vi "ADCP_read_parameter_from_serial_port_Test.vi"() -> ()   [LabVIEW 2017]
uses:
  Classes/ADCP.lvclass
panel:
  in  "Stop Application":bool
  out "Parameter Value":string
  in  "Parameter to monitor":string(combo)
  in  "Symbol File Path":path
  in  "ADCP Session Parameters":T1
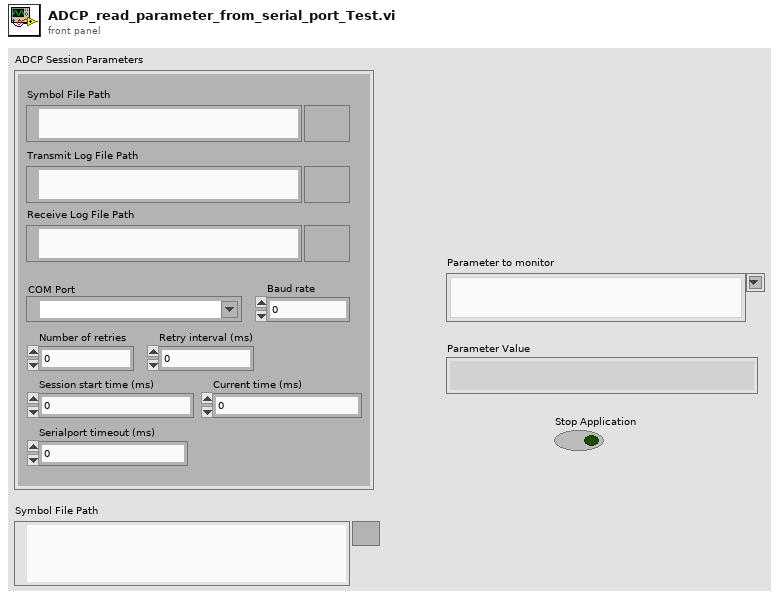
[diagram p1: front panel]
types:
  T1 = cluster{"Symbol File Path":path, "Transmit Log File Path":path, "Receive Log File Path":path, "COM Port":refnum<visa-resource-name>, "Baud rate":u32, "Number of retries":u16, "Retry interval (ms)":u16, "Session start time (ms)":u32, "Current time (ms)":u32, "Serialport timeout (ms)":u32}
  T2 = typedef "ADCP.lvclass/ADCP_Packet_Info.ctl" = cluster{"Priority":enum16{"LOW", "HIGH"}, "Type":enum16{"Data", "Connection Management", "Remote Request", "Error and status", "INVALID"}, "Node ID":i32, "Frame ID":i32, "Checksum valid ?":bool, "Current time (ms)":u32}
  T3 = enum16{"Data", "Connection Management", "Remote Request", "Error and status", "INVALID"}
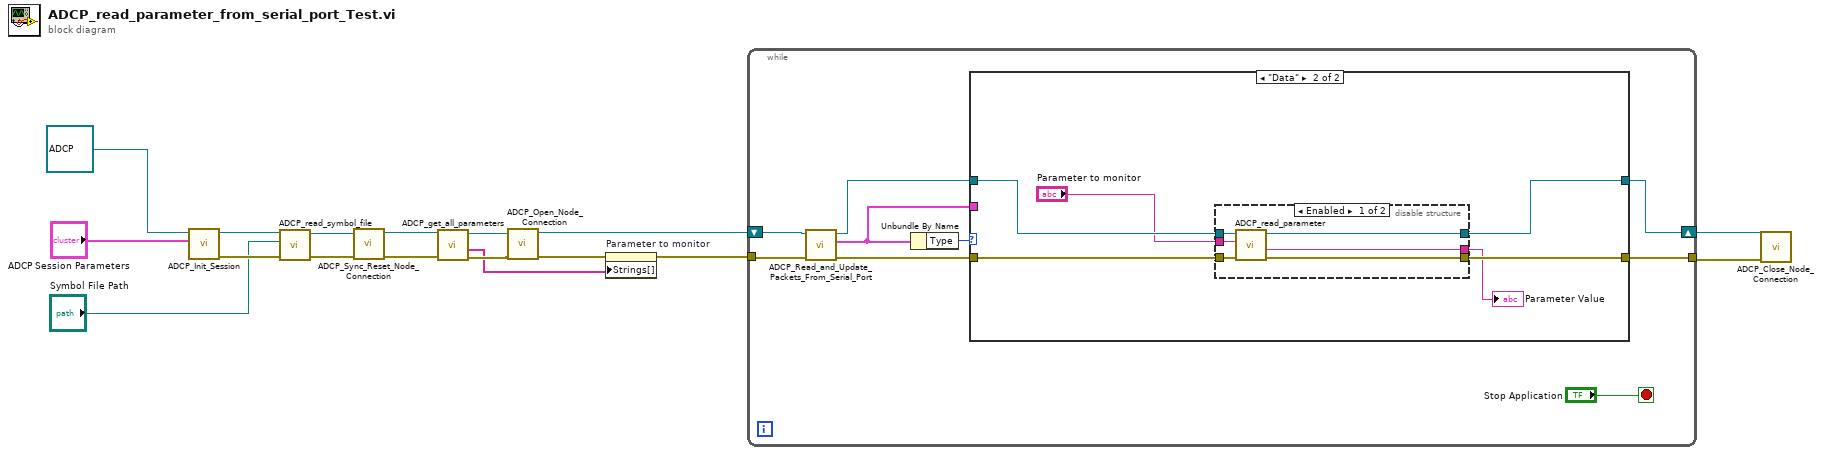
[diagram p0: block diagram]
diagram:
  n1 = call "ADCP_Init_Session.vi"("ADCP Session Parameters"="ADCP Session Parameters", "ADCP in"=refnum<class "ADCP.lvclass"> refnum) -> ("error out"=w15:errorcluster, "ADCP out"=w16:refnum<class "ADCP.lvclass">)  [unwired: 8 in]
  n2 = call "ADCP_read_symbol_file.vi"("error in (no error)"=w15, "Symbol File Path"="Symbol File Path", "ADCP in"=w16) -> ("error out"=w2:errorcluster, "ADCP out"=w4:refnum<class "ADCP.lvclass">)  [unwired: 5 in, 2 out]
  n3 = call "ADCP_Sync_Reset_Node_Connection.vi"("error in (no error)"=w2, "ADCP In"=w4) -> ("error out"=w1:errorcluster, "ADCP Out"=w3:refnum<class "ADCP.lvclass">)  [unwired: 8 in]
  n4 = call "ADCP_get_all_parameters.vi"("error in (no error)"=w1, "ADCP In"=w3) -> ("error out"=w12:errorcluster, "Parameter names"=w9:string[], "ADCP Out"=w13:refnum<class "ADCP.lvclass">)  [unwired: 6 in, 1 out]
  n5 = call "ADCP_Open_Node_Connection.vi"("error in (no error)"=w12, "ADCP In"=w13) -> ("error out"=w10:errorcluster, "ADCP Out"=w11:refnum<class "ADCP.lvclass">)  [unwired: 8 in]
  n6 = property on="Parameter to monitor" class="CmbBox"(error in=w10, "Strings[]"=w9) -> (error out=w8:errorcluster)  [unwired: 1 in, 1 out]
  n7 = while {
    tunnel: w8 -> [w25]
    shift-right: [w20] -> w7
    shift-left: w11 -> [w26]
    tunnel: [w19] -> w6
    stop <- "Stop Application" stop-if-true
    n8 = call "ADCP_Read_and_Update_Packets_From_Serial_Port.vi"("error in (no error)"=w25, "ADCP In"=w26) -> ("error out"=w22:errorcluster, "Packet Info"=w21:T2, "ADCP out"=w23:refnum<class "ADCP.lvclass">)  [unwired: 6 in, 1 out]
    n9 = Unbundle By Name(w21) -> ("Type"=w24:T3)
    n10 = case shown="\"Data\"" w24 {
      tunnel: w23 -> [w28 w33]
      tunnel: w22 -> [w27 w34]
      tunnel: w21 -> [_ _]
      tunnel: [w28 w32] -> w20
      tunnel: [w27 w31] -> w19
      frame Default {
      }
      frame "Data" {
        n11 = disable-structure shown="Enabled" {
          disable-tunnel: w34 -> [w40 w41]
          disable-tunnel: w33 -> [w39 w42]
          disable-tunnel: [w38 w42] -> w32
          disable-tunnel: [w37 w41] -> w31
          disable-tunnel: [w36 _] -> w30
          disable-tunnel: "Parameter to monitor" -> [w35 _]
          frame Enabled {
            n12 = call "ADCP_read_parameter.vi"("error in (no error)"=w40, "Parameter Name"=w35, "ADCP In"=w39) -> ("error out"=w37:errorcluster, "Parameter Value"=w36:string, "ADCP out"=w38:refnum<class "ADCP.lvclass">)  [unwired: 5 in, 1 out]
          }
          frame Disabled {
          }
        }
        "Parameter Value" <- w30
      }
    }
  }
  n13 = call "ADCP_Close_Node_Connection.vi"("error in (no error)"=w6, "ADCP In"=w7) -> ()  [unwired: 8 in, 2 out]
